vi "JSON text to Variant.vi"(6 "LVClass Serializer":refnum<class "JSONtext LVClass Serializer.lvclass">, 8 "error in (no error)":errorcluster, 9 "Data Type":variant, 10 "Offset":i32, 11 "JSON":string) -> (0 "error out":errorcluster, 1 "Variant out":variant)   [LabVIEW 2019, in "JSONtext.lvlib"]
doc: "Convert JSON to the Data Type entered, which may be a cluster or array."
uses:
  JSONtext.lvlib
  LVClass Serializer/JSONtext LVClass Serializer.lvclass
  <vilib>/Utility/Data Type/Type Definitions/Data Type.ctl
  Parsing/Advance past Line Ending.vi
  support/Get String.vi
  support/Get Timestamp.vi
  support/Get I32.vi
  support/Get I64.vi
  support/Get U32.vi
  support/Get U64.vi
  support/Get Boolean.vi
  support/Get DBL.vi
  support/Get SGL.vi
  support/Unescape JSON string.vi
  support/quote and escape json string 2.vi
  Parsing/Advance past whitespace and comma.vi
  Parsing/Advance past next JSON Value (inlined COPY).vi
  Parsing/Advance past Item Name.vi
  Base64/base64url Decode.vi
  Parsing/Advance past String.vi
  support/Get Number Text.vi
  Parsing/NaN or null to Integer ERROR.vi
  Parsing/Advance past Number.vi
  <vilib>/Utility/error.llb/Error Cluster From Error Code.vi
  <vilib>/Utility/Data Type/Get Refnum Information.vi
  support/Error Cluster From Code.vi
  JDP Science Common Utilities/Timestamp/Text to Timestamp.vi
  <vilib>/Utility/Data Type/Get Numeric Information.vi
  Parsing/Advance past Object.vi
  Parsing/Parsing Error.vi
  <vilib>/Utility/Data Type/NI_Data Type.lvlib
  JDP Science Common Utilities/JDP Utility.lvlib
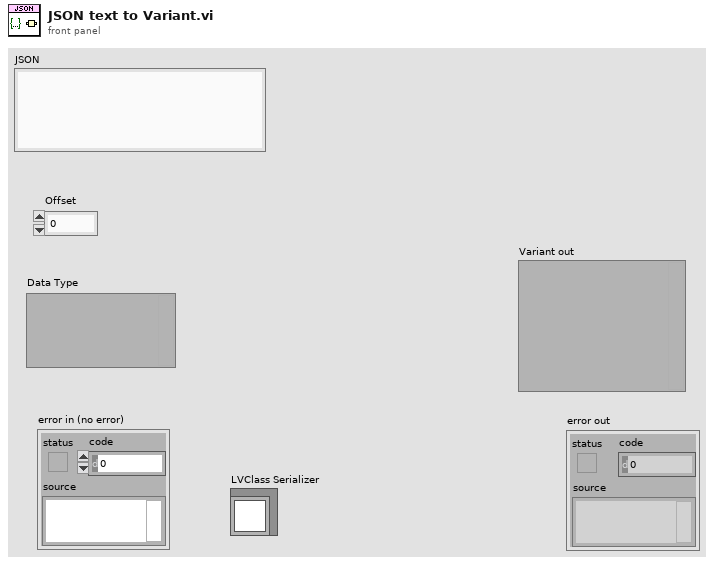
[diagram p1: front panel]
types:
  T1 = typedef "NI_Data Type.lvlib/Data Type.ctl" = enum8{"Invalid Type", "Void", "I8", "I16", "I32", "I64", "U8", "U16", "U32", "U64", "Single Float", "Double Float", "Extended Float", "Single Complex", "Double Complex", "Extended Complex", "Enum U8", "Enum U16", "Enum U32", "Enum U64", "Single Float With Unit", "Double Float With Unit", "Extended Float With Unit", "Single Complex with Unit", "Double Complex with Unit", "Extended Complex with Unit", "Boolean", "String", "Path", "Picture", "Tag", "Array", "Cluster", "Variant", "LV Variant", "Waveform", "Timestamp", "Digital Waveform", "Digital Data", "ExpressData", "Refnum", "External Data", "VI", "Poly VI", "LabVIEW Class Instance", "Fixed Point", "Set Collection", "Map Collection"}
  T2 = typedef "JSONtext.lvlib/Parsing State.ctl" = enum16{"Parser Error", "Object", "Array", "String", "Number/Other", "Leading Whitespace", "Object end", "Array end", "Value end"}
  T3 = typedef "JSONtext.lvlib/Tag Type.ctl" = enum16{"No Tag", "<JSON>", "<JOBJ>"}
  T4 = typedef "JSONtext.lvlib/JSON Value Type.ctl" = enum16{"Not a JSON Value", "JSON Object", "JSON Array", "String", "Number", "true", "false", "null"}
  T5 = typedef "JSONtext.lvlib/Found Items.ctl" = cluster{"Item offset":i32, "Offset past Item":i32, "Name offset":i32, "Offset past Name":i32, "Found":bool, "Item Type":T2, "Item Index":i32, "Start Offset":i32, "Comma Needed For Insert":bool}
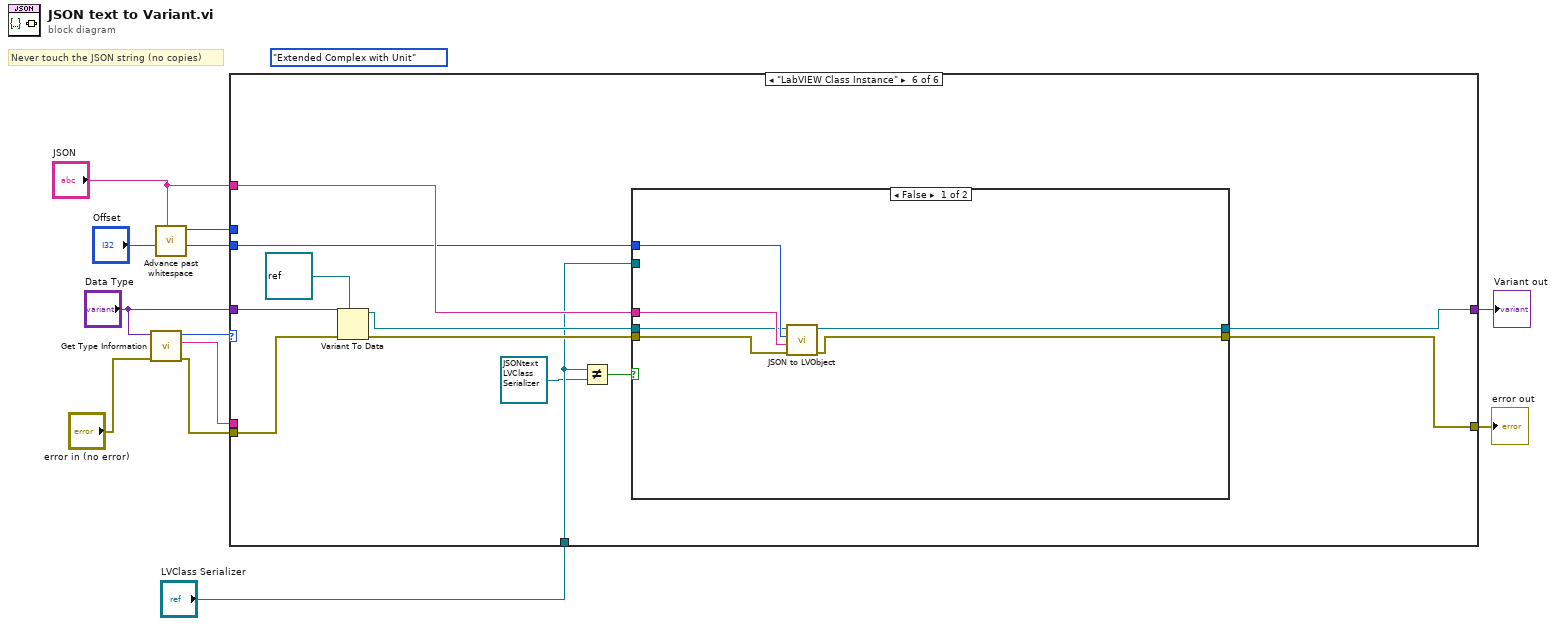
[diagram p0: block diagram]
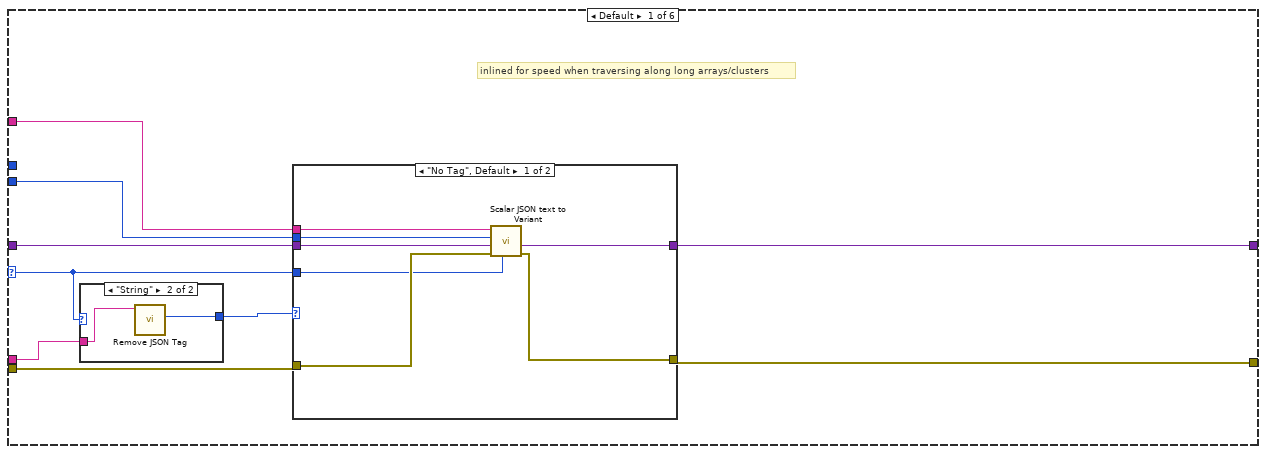
[diagram p2: hidden frame]
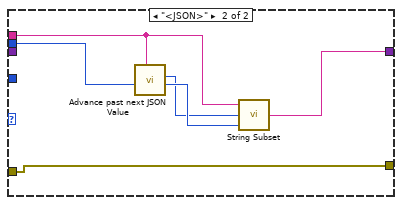
[diagram p3: hidden frame]
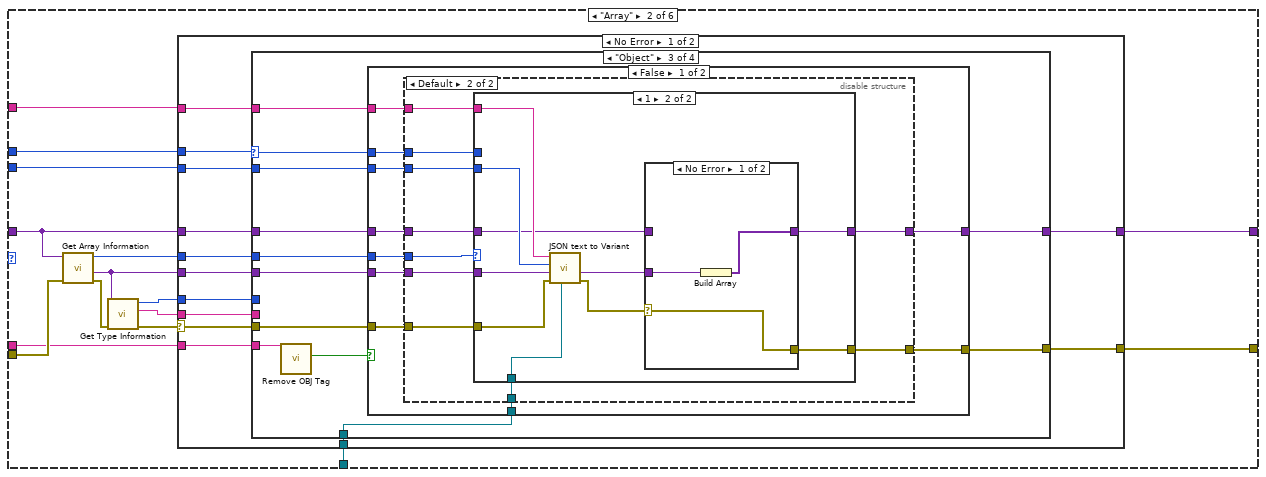
[diagram p5: hidden frame]
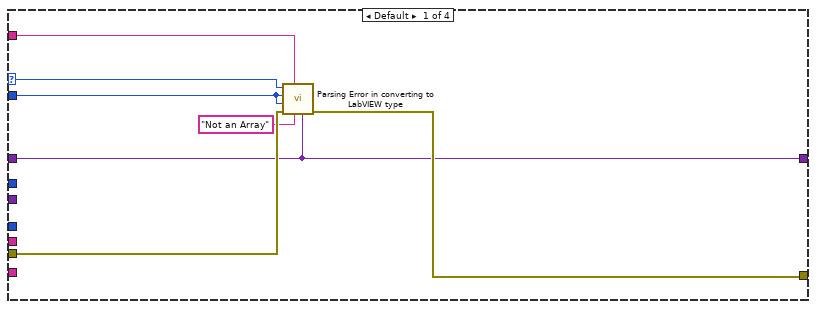
[diagram p6: hidden frame]
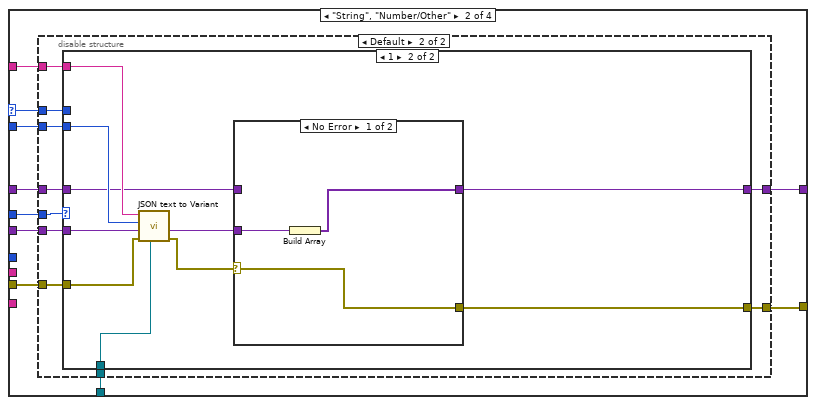
[diagram p7: hidden frame]
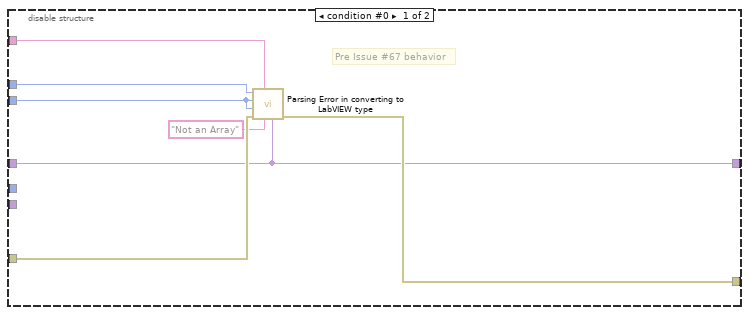
[diagram p8: hidden frame]
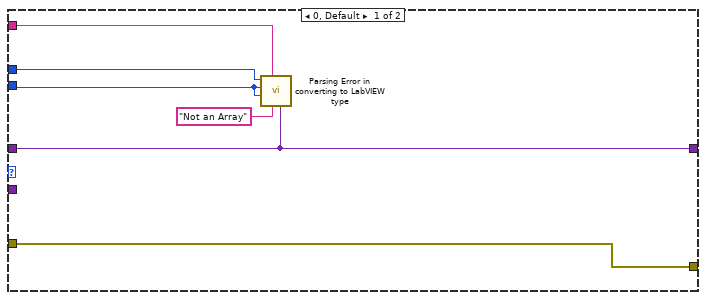
[diagram p9: hidden frame]
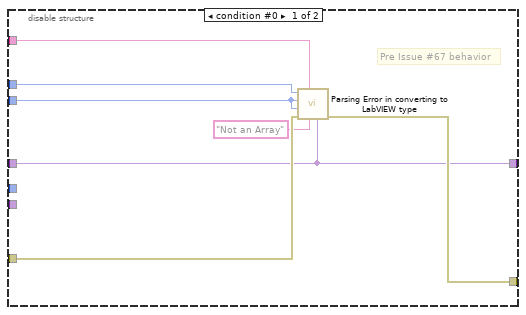
[diagram p11: hidden frame]
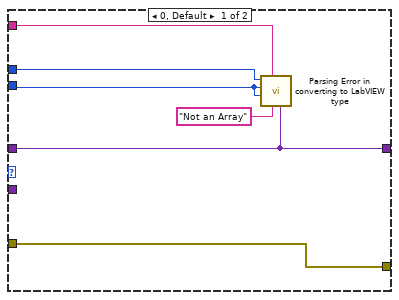
[diagram p12: hidden frame]
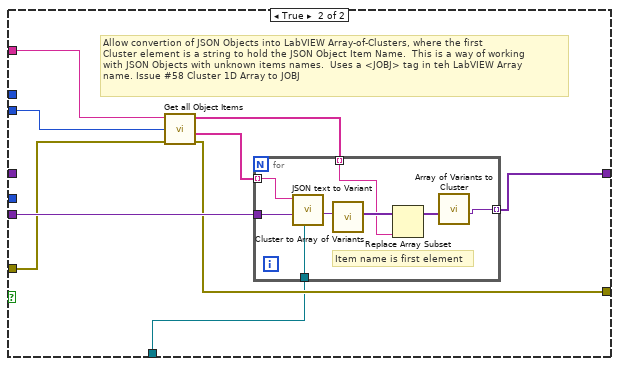
[diagram p14: hidden frame]
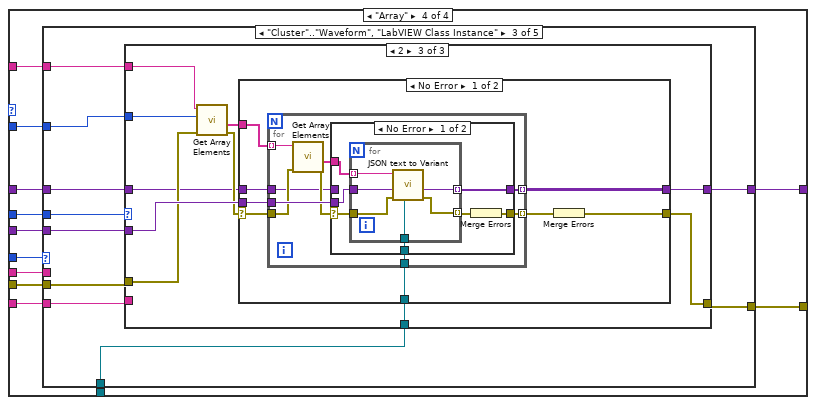
[diagram p15: hidden frame]
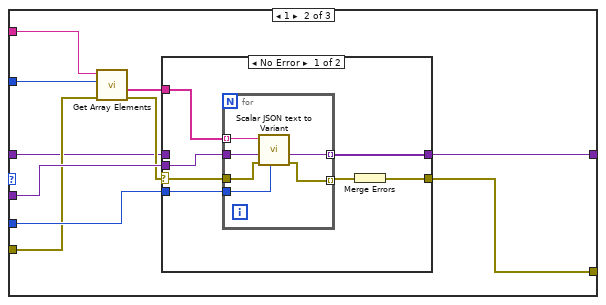
[diagram p18: hidden frame]
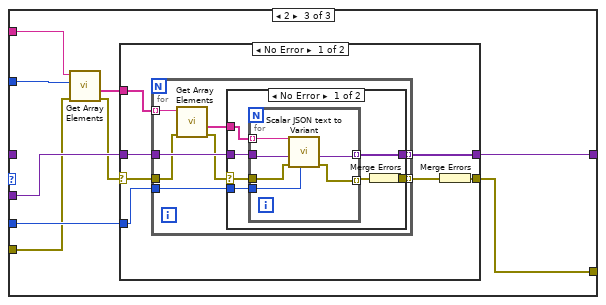
[diagram p20: hidden frame]
diagram:
  (unwired) Data_Type."Extended Complex with Unit" ("Type")
  # "Never touch the JSON string (no copies)"
  n1 = call <vilib>:"Get Type Information.vi"("error in (no error)"="error in (no error)", "variant"="Data Type") -> ("error out"=w8:errorcluster, "name"=w2:string, "type"=w12:T1)  [unwired: 5 in, 2 out]
  n2 = call "Advance past whitespace.vi"("JSON"="JSON", "Offset"="Offset") -> ("Offset of first non-whitespace"=w5:i32, "Parser State"=w3:T2)  [unwired: 7 in, 1 out]
  n3 = case shown="\"LabVIEW Class Instance\"" w12 {
    selector: w12 -> [w14 _ _ _ _ _]
    tunnel: "Data Type" -> [w21 w44 w586 w595 w795 w806]
    tunnel: "JSON" -> [w19 w42 w579 w591 w790 w807]
    tunnel: [w16 w48 w576 w593 w787 w800] -> w9
    tunnel: w8 -> [w17 w51 w585 w594 w794 w804]
    tunnel: w5 -> [w18 w40 w578 w592 w789 w799]
    tunnel: [w20 w47 w569 w588 w792 w801] -> w7
    tunnel: w3 -> [_ w38 _ _ _ _]
    tunnel: w2 -> [w15 w41 _ _ _ _]
    tunnel: "LVClass Serializer" -> [_ w37 w568 w587 w785 w798]
    frame Default {
      # "inlined for speed when traversing along long arrays/clusters"
      n4 = case shown="\"String\"" w14 {
        tunnel: w15 -> [_ w36]
        tunnel: [_ w35] -> w13
        frame "Invalid Type", Default {
        }
        frame "String" {
          n5 = call "Remove JSON Tag.vi"("Name"=w36) -> ("Tag"=w35:T3)  [unwired: 9 in, 1 out]
        }
      }
      n6 = case shown="\"No Tag\", Default" w13 {
        tunnel: w21 -> [w28 _]
        tunnel: [w27 w30] -> w20
        tunnel: w19 -> [w26 w31]
        tunnel: w18 -> [w25 w34]
        tunnel: w17 -> [w24 w29]
        tunnel: [w23 w29] -> w16
        tunnel: w14 -> [w22 _]
        frame "No Tag", Default {
          n7 = call "Scalar JSON text to Variant.vi"("Type"=w22, "error in (no error)"=w24, "Variant (Data Type)"=w28, "Offset"=w25, "JSON"=w26) -> ("error out"=w23:errorcluster, "Variant out"=w27:variant)  [unwired: 5 in]
        }
        frame "<JSON>" {
          n8 = call "Advance past next JSON Value.vi"("JSON"=w31, "Offset"=w34) -> ("Offset out"=w33:i32, "Value start"=w32:i32)  [unwired: 7 in, 1 out]
          n9 = call "String Subset.vi"("Offset past End"=w33, "Start offset"=w32, "JSON"=w31) -> ("substring"=w30:string)  [unwired: 2 in]
        }
      }
    }
    frame "Array" {
      n10 = call <vilib>:"Get Array Information.vi"("error in (no error)"=w51, "variant"=w44) -> ("error out"=w50:errorcluster, "array element data type"=w43:variant, "number of dimensions"=w45:i32)  [unwired: 6 in, 1 out]
      n11 = call <vilib>:"Get Type Information.vi"("error in (no error)"=w50, "variant"=w43) -> ("error out"=w49:errorcluster, "name"=w39:string, "type"=w46:T1)  [unwired: 5 in, 2 out]
      n12 = case shown="No Error" w49 {
        selector: w49 -> [w64 w567]
        tunnel: [w63 w567] -> w48
        tunnel: [w62 w566] -> w47
        tunnel: w46 -> [w61 _]
        tunnel: w45 -> [w60 _]
        tunnel: w44 -> [w59 w566]
        tunnel: w43 -> [w58 _]
        tunnel: w42 -> [w57 _]
        tunnel: w41 -> [w56 _]
        tunnel: w40 -> [w55 _]
        tunnel: w39 -> [w54 _]
        tunnel: w38 -> [w53 _]
        tunnel: w37 -> [w52 _]
        frame No Error {
          n13 = case shown="\"Object\"" w53 {
            selector: w53 -> [w69 w79 w129 _]
            tunnel: w64 -> [w68 w78 w128 w208]
            tunnel: [w67 w77 w127 w207] -> w63
            tunnel: [w66 w74 w124 w206] -> w62
            tunnel: w61 -> [_ _ _ w205]
            tunnel: w60 -> [_ w73 w123 w204]
            tunnel: w59 -> [w66 w76 w126 w203]
            tunnel: w58 -> [_ w75 w125 w202]
            tunnel: w57 -> [w71 w81 w131 w201]
            tunnel: w56 -> [_ _ w121 w200]
            tunnel: w55 -> [w70 w80 w130 w199]
            tunnel: w54 -> [_ _ _ w198]
            tunnel: w52 -> [_ w72 w122 w197]
            frame Default {
              n14 = call "Parsing Error in converting to LabVIEW type.vi"("LV Type"=w66, "initial string"="Not an Array", "JSON"=w71, "error in (no error)"=w68, "Offset past match"=w70, "Value start"=w70, "State"=w69) -> ("error out"=w67:errorcluster)  [unwired: 4 in]
            }
            frame "String", "Number/Other" {
              n15 = disable-structure shown="Default" {
                disable-tunnel: w81 -> [w88 w97]
                disable-tunnel: w80 -> [w87 w96]
                disable-tunnel: w79 -> [w86 w90]
                disable-tunnel: w78 -> [w85 w95]
                disable-tunnel: [w84 w92] -> w77
                disable-tunnel: w76 -> [w82 w93]
                disable-tunnel: w75 -> [_ w98]
                disable-tunnel: [w82 w94] -> w74
                disable-tunnel: w73 -> [_ w91]
                disable-tunnel: w72 -> [_ w89]
                frame condition #0 {
                  # "Pre Issue #67 behavior"
                  n16 = call "Parsing Error in converting to LabVIEW type.vi"("LV Type"=w82, "initial string"="Not an Array", "JSON"=w88, "error in (no error)"=w85, "Offset past match"=w87, "Value start"=w87, "State"=w86) -> ("error out"=w84:errorcluster)  [unwired: 4 in]
                }
                frame condition #1 (active) {
                  n17 = case shown="1" w91 {
                    tunnel: w98 -> [_ w114]
                    tunnel: w97 -> [w103 w113]
                    tunnel: w96 -> [w101 w112]
                    tunnel: w95 -> [w99 w110]
                    tunnel: [w100 w108] -> w94
                    tunnel: w93 -> [w100 w107]
                    tunnel: [w99 w106] -> w92
                    tunnel: w90 -> [w102 _]
                    tunnel: w89 -> [_ w105]
                    frame 0, Default {
                      n18 = call "Parsing Error in converting to LabVIEW type.vi"("LV Type"=w100, "initial string"="Not an Array", "JSON"=w103, "Offset past match"=w101, "Value start"=w101, "State"=w102) -> ()  [unwired: 5 in, 1 out]
                    }
                    frame 1 {
                      n19 = call "JSON text to Variant.vi"("LVClass Serializer"=w105, "error in (no error)"=w110, "Data Type"=w114, "Offset"=w112, "JSON"=w113) -> ("error out"=w109:errorcluster, "Variant out"=w111:variant)  [unwired: 5 in]
                      n20 = case shown="No Error" w109 {
                        selector: w109 -> [w115 w118]
                        tunnel: w111 -> [w117 _]
                        tunnel: [w116 w119] -> w108
                        tunnel: w107 -> [_ w119]
                        tunnel: [w115 w118] -> w106
                        frame No Error {
                          n21 = Build Array(w117) -> (w116:variant[])
                        }
                        frame Error {
                        }
                      }
                    }
                  }
                }
              }
            }
            frame "Object" {
              n22 = call "Remove OBJ Tag.vi"("Name"=w121) -> ("tagged as Item Name in JSON Objects"=w120:bool)  [unwired: 9 in, 1 out]
              n23 = case shown="False" w120 {
                tunnel: w131 -> [w141 w186]
                tunnel: w130 -> [w140 w180]
                tunnel: w129 -> [w139 _]
                tunnel: w128 -> [w138 w187]
                tunnel: [w137 w184] -> w127
                tunnel: w126 -> [w136 _]
                tunnel: w125 -> [w135 w188]
                tunnel: [w134 w185] -> w124
                tunnel: w123 -> [w133 _]
                tunnel: w122 -> [w132 w183]
                frame False {
                  n24 = disable-structure shown="Default" {
                    disable-tunnel: w141 -> [w148 w157]
                    disable-tunnel: w140 -> [w147 w156]
                    disable-tunnel: w139 -> [w146 w150]
                    disable-tunnel: w138 -> [w145 w155]
                    disable-tunnel: [w144 w152] -> w137
                    disable-tunnel: w136 -> [w142 w153]
                    disable-tunnel: w135 -> [_ w158]
                    disable-tunnel: [w142 w154] -> w134
                    disable-tunnel: w133 -> [_ w151]
                    disable-tunnel: w132 -> [_ w149]
                    frame condition #0 {
                      # "Pre Issue #67 behavior"
                      n25 = call "Parsing Error in converting to LabVIEW type.vi"("LV Type"=w142, "initial string"="Not an Array", "JSON"=w148, "error in (no error)"=w145, "Offset past match"=w147, "Value start"=w147, "State"=w146) -> ("error out"=w144:errorcluster)  [unwired: 4 in]
                    }
                    frame condition #1 (active) {
                      n26 = case shown="1" w151 {
                        tunnel: w158 -> [_ w174]
                        tunnel: w157 -> [w163 w173]
                        tunnel: w156 -> [w161 w172]
                        tunnel: w155 -> [w159 w170]
                        tunnel: [w160 w168] -> w154
                        tunnel: w153 -> [w160 w167]
                        tunnel: [w159 w166] -> w152
                        tunnel: w150 -> [w162 _]
                        tunnel: w149 -> [_ w165]
                        frame 0, Default {
                          n27 = call "Parsing Error in converting to LabVIEW type.vi"("LV Type"=w160, "initial string"="Not an Array", "JSON"=w163, "Offset past match"=w161, "Value start"=w161, "State"=w162) -> ()  [unwired: 5 in, 1 out]
                        }
                        frame 1 {
                          n28 = call "JSON text to Variant.vi"("LVClass Serializer"=w165, "error in (no error)"=w170, "Data Type"=w174, "Offset"=w172, "JSON"=w173) -> ("error out"=w169:errorcluster, "Variant out"=w171:variant)  [unwired: 5 in]
                          n29 = case shown="No Error" w169 {
                            selector: w169 -> [w175 w178]
                            tunnel: w171 -> [w177 _]
                            tunnel: [w176 w179] -> w168
                            tunnel: w167 -> [_ w179]
                            tunnel: [w175 w178] -> w166
                            frame No Error {
                              n30 = Build Array(w177) -> (w176:variant[])
                            }
                            frame Error {
                            }
                          }
                        }
                      }
                    }
                  }
                }
                frame True {
                  # "Allow convertion of JSON Objects into LabVIEW Array-of-Clusters, where the first\nCluster element is a string to hold the JSON Object Item Name.  This is a way of working\nwith JSON Objects with unknown items names.  Uses a <JOBJ> tag in teh LabVIEW Array\nname. Issue #58 Cluster 1D Array to JOBJ"
                  n31 = call "Get all Object Items.vi"("error in (no error)"=w187, "Offset"=w180, "JSON"=w186) -> ("error out"=w184:errorcluster, "<JSON>"=w182:string[], "Item Names"=w181:string[])  [unwired: 5 in, 1 out]
                  n32 = for {
                    tunnel: w182 -> [w196] mode=indexing
                    tunnel: w188 -> [w195]
                    tunnel: w181 -> [w191] mode=indexing
                    tunnel: [w190] -> w185 mode=indexing
                    tunnel: w183 -> [w189]
                    # "Item name is first element"
                    n33 = call "JSON text to Variant.vi"("LVClass Serializer"=w189, "Data Type"=w195, "JSON"=w196) -> ("Variant out"=w193:variant)  [unwired: 7 in, 1 out]
                    n34 = call "Cluster to Array of Variants.vi"("Cluster"=w193) -> ("Array of Cluster Elements"=w192:variant[])  [unwired: 10 in]
                    n35 = Replace Array Subset(array=w192, new element=w191) -> (w194:variant[])  [unwired: 1 in]
                    n36 = call "Array of Variants to Cluster.vi"("Array of Variants"=w194) -> ("Cluster of Variants"=w190:variant)  [unwired: 10 in]
                  }
                }
              }
            }
            frame "Array" {
              n37 = case shown="\"Cluster\"..\"Waveform\", \"LabVIEW Class Instance\"" w205 {
                selector: w205 -> [_ w211 _ w375 _]
                tunnel: w201 -> [_ w215 w293 w373 w503]
                tunnel: w208 -> [w209 w218 w296 w380 w502]
                tunnel: [w209 w219 w297 w379 w501] -> w207
                tunnel: [w210 w216 w294 w378 w500] -> w206
                tunnel: w204 -> [_ w214 w292 w377 w499]
                tunnel: w203 -> [w210 w213 w291 w376 w498]
                tunnel: w202 -> [_ w217 w295 _ _]
                tunnel: w199 -> [_ w212 w290 w372 w496]
                tunnel: w200 -> [_ _ w289 _ w497]
                tunnel: w198 -> [_ _ _ _ w495]
                tunnel: w197 -> [_ _ w288 _ _]
                frame "Invalid Type" {
                }
                frame Default {
                  # "Scaler type (so we are using the inlined function"
                  n38 = case shown="0, Default" w214 {
                    tunnel: [w220 w231 w250] -> w219
                    tunnel: w218 -> [w220 w224 w248]
                    tunnel: w217 -> [_ w230 w255]
                    tunnel: [w221 w228 w253] -> w216
                    tunnel: w212 -> [_ w227 w252]
                    tunnel: w215 -> [_ w226 w251]
                    tunnel: w213 -> [w221 w222 _]
                    tunnel: w211 -> [_ w225 w249]
                    frame 0, Default {
                    }
                    frame 1 {
                      n39 = call "Get Array Elements.vi"("error in (no error)"=w224, "Offset"=w227, "JSON"=w226) -> ("error out"=w223:errorcluster, "<JSON>"=w229:string[])  [unwired: 6 in, 1 out]
                      n40 = case shown="No Error" w223 {
                        selector: w223 -> [w232 w245]
                        tunnel: [w237 w245] -> w231
                        tunnel: w230 -> [w236 _]
                        tunnel: w229 -> [w235 _]
                        tunnel: [w234 w246] -> w228
                        tunnel: w225 -> [w233 _]
                        tunnel: w222 -> [_ w246]
                        frame No Error {
                          n41 = for {
                            tunnel: w236 -> [w243]
                            tunnel: w232 -> [w241]
                            tunnel: [w240] -> w238 mode=indexing
                            tunnel: [w242] -> w234 mode=indexing
                            tunnel: w235 -> [w244] mode=indexing
                            tunnel: w233 -> [w239]
                            n42 = call "Scalar JSON text to Variant.vi"("Type"=w239, "error in (no error)"=w241, "Variant (Data Type)"=w243, "JSON"=w244) -> ("error out"=w240:errorcluster, "Variant out"=w242:variant)  [unwired: 6 in]
                          }
                          n43 = Merge Errors(w238) -> (w237:errorcluster)
                        }
                        frame Error {
                        }
                      }
                    }
                    frame 2 {
                      n44 = call "Get Array Elements.vi"("error in (no error)"=w248, "Offset"=w252, "JSON"=w251) -> ("error out"=w247:errorcluster, "<JSON>"=w254:string[])  [unwired: 6 in, 1 out]
                      n45 = case shown="No Error" w247 {
                        selector: w247 -> [w256 w287]
                        tunnel: w255 -> [w261 w286]
                        tunnel: w254 -> [w260 _]
                        tunnel: [w259 w286] -> w253
                        tunnel: [w258 w287] -> w250
                        tunnel: w249 -> [w257 _]
                        frame No Error {
                          n46 = for {
                            tunnel: [w270] -> w262 mode=indexing
                            tunnel: w256 -> [w264]
                            tunnel: w261 -> [w269]
                            tunnel: w260 -> [w267] mode=indexing
                            tunnel: [w268] -> w259 mode=indexing
                            tunnel: w257 -> [w265]
                            n47 = call "Get Array Elements.vi"("error in (no error)"=w264, "JSON"=w267) -> ("error out"=w263:errorcluster, "<JSON>"=w266:string[])  [unwired: 7 in, 1 out]
                            n48 = case shown="No Error" w263 {
                              selector: w263 -> [w271 w284]
                              tunnel: [w276 w284] -> w270
                              tunnel: w269 -> [w275 w285]
                              tunnel: [w274 w285] -> w268
                              tunnel: w266 -> [w273 _]
                              tunnel: w265 -> [w272 _]
                              frame No Error {
                                n49 = for {
                                tunnel: w275 -> [w279]
                                tunnel: w271 -> [w280]
                                tunnel: [w281] -> w277 mode=indexing
                                tunnel: [w282] -> w274 mode=indexing
                                tunnel: w273 -> [w283] mode=indexing
                                tunnel: w272 -> [w278]
                                n50 = call "Scalar JSON text to Variant.vi"("Type"=w278, "error in (no error)"=w280, "Variant (Data Type)"=w279, "JSON"=w283) -> ("error out"=w281:errorcluster, "Variant out"=w282:variant)  [unwired: 6 in]
                                }
                                n51 = Merge Errors(w277) -> (w276:errorcluster)
                              }
                              frame Error {
                              }
                            }
                          }
                          n52 = Merge Errors(w262) -> (w258:errorcluster)
                        }
                        frame Error {
                        }
                      }
                    }
                  }
                }
                frame "Cluster".."Waveform", "LabVIEW Class Instance" {
                  n53 = case shown="2" w292 {
                    tunnel: [w298 w309 w329] -> w297
                    tunnel: w296 -> [w298 w308 w328]
                    tunnel: w295 -> [_ w307 w334]
                    tunnel: [w299 w306 w332] -> w294
                    tunnel: w290 -> [_ w304 w331]
                    tunnel: w293 -> [_ w305 w330]
                    tunnel: w291 -> [w299 w303 w326]
                    tunnel: w289 -> [_ _ _]
                    tunnel: w288 -> [_ w302 w325]
                    frame 0, Default {
                    }
                    frame 1 {
                      n54 = call "Get Array Elements.vi"("error in (no error)"=w308, "Offset"=w304, "JSON"=w305) -> ("error out"=w300:errorcluster, "<JSON>"=w301:string[])  [unwired: 6 in, 1 out]
                      n55 = case shown="No Error" w300 {
                        selector: w300 -> [w311 w324]
                        tunnel: [w315 w324] -> w309
                        tunnel: w307 -> [w314 _]
                        tunnel: [w313 w323] -> w306
                        tunnel: w301 -> [w312 _]
                        tunnel: w303 -> [_ w323]
                        tunnel: w302 -> [w310 _]
                        frame No Error {
                          n56 = for {
                            tunnel: w314 -> [w322]
                            tunnel: w311 -> [w321]
                            tunnel: [w320] -> w316 mode=indexing
                            tunnel: [w319] -> w313 mode=indexing
                            tunnel: w312 -> [w318] mode=indexing
                            tunnel: w310 -> [w317]
                            n57 = call "JSON text to Variant.vi"("LVClass Serializer"=w317, "error in (no error)"=w321, "Data Type"=w322, "JSON"=w318) -> ("error out"=w320:errorcluster, "Variant out"=w319:variant)  [unwired: 6 in]
                          }
                          n58 = Merge Errors(w316) -> (w315:errorcluster)
                        }
                        frame Error {
                        }
                      }
                    }
                    frame 2 {
                      n59 = call "Get Array Elements.vi"("error in (no error)"=w328, "Offset"=w331, "JSON"=w330) -> ("error out"=w327:errorcluster, "<JSON>"=w333:string[])  [unwired: 6 in, 1 out]
                      n60 = case shown="No Error" w327 {
                        selector: w327 -> [w337 w369]
                        tunnel: w334 -> [w341 _]
                        tunnel: w333 -> [w340 _]
                        tunnel: [w339 w368] -> w332
                        tunnel: [w338 w369] -> w329
                        tunnel: w326 -> [w336 w368]
                        tunnel: w325 -> [w335 _]
                        frame No Error {
                          n61 = for {
                            tunnel: [w351] -> w342 mode=indexing
                            tunnel: w337 -> [w346]
                            tunnel: w341 -> [w350]
                            tunnel: w340 -> [w348] mode=indexing
                            tunnel: [w349] -> w339 mode=indexing
                            tunnel: w336 -> [w344]
                            tunnel: w335 -> [w343]
                            n62 = call "Get Array Elements.vi"("error in (no error)"=w346, "JSON"=w348) -> ("error out"=w345:errorcluster, "<JSON>"=w347:string[])  [unwired: 7 in, 1 out]
                            n63 = case shown="No Error" w345 {
                              selector: w345 -> [w353 w367]
                              tunnel: [w357 w367] -> w351
                              tunnel: w350 -> [w356 w365]
                              tunnel: [w355 w366] -> w349
                              tunnel: w347 -> [w354 _]
                              tunnel: w344 -> [_ _]
                              tunnel: w343 -> [w352 _]
                              frame No Error {
                                n64 = for {
                                tunnel: w356 -> [w364]
                                tunnel: w353 -> [w363]
                                tunnel: [w362] -> w358 mode=indexing
                                tunnel: [w361] -> w355 mode=indexing
                                tunnel: w354 -> [w360] mode=indexing
                                tunnel: w352 -> [w359]
                                n65 = call "JSON text to Variant.vi"("LVClass Serializer"=w359, "error in (no error)"=w363, "Data Type"=w364, "JSON"=w360) -> ("error out"=w362:errorcluster, "Variant out"=w361:variant)  [unwired: 6 in]
                                }
                                n66 = Merge Errors(w358) -> (w357:errorcluster)
                              }
                              frame Error {
                                n67 = Build Array(w365) -> (w366:variant[])
                              }
                            }
                          }
                          n68 = Merge Errors(w342) -> (w338:errorcluster)
                        }
                        frame Error {
                        }
                      }
                    }
                  }
                }
                frame "I8".."Extended Complex", "Single Float With Unit".."Extended Float With Unit" {
                  # "Use LV JSON primative for speed"
                  n69 = call "Advance past Array.vi"("JSON"=w373, "Offset"=w372) -> ("Offset past Array"=w374:i32, "Empty Array"=w370:bool, "Array Start"=w371:i32)  [unwired: 6 in, 1 out]
                  n70 = case shown="False" w370 {
                    tunnel: w380 -> [w390 w493]
                    tunnel: [w389 w493] -> w379
                    tunnel: [w388 w492] -> w378
                    tunnel: w377 -> [w387 _]
                    tunnel: w376 -> [w386 w492]
                    tunnel: w375 -> [w384 _]
                    tunnel: w374 -> [w383 _]
                    tunnel: w373 -> [w382 _]
                    tunnel: w371 -> [w381 _]
                    frame False {
                      n71 = call "String Subset.vi"("Offset past End"=w383, "Start offset"=w381, "JSON"=w382) -> ("substring"=w385:string)  [unwired: 2 in]
                      n72 = case shown="0, Default" w387 {
                        tunnel: w385 -> [_ w398 w431 w464]
                        tunnel: w390 -> [w391 w397 w430 w463]
                        tunnel: [w391 w396 w429 w462] -> w389
                        tunnel: [w392 w394 w427 w460] -> w388
                        tunnel: w386 -> [w392 w393 w426 w459]
                        tunnel: w384 -> [_ w395 w428 w461]
                        frame 0, Default {
                        }
                        frame 1 {
                          n73 = case shown="\"I8\"..\"I32\"" w395 {
                            tunnel: w398 -> [_ w405 w410 w415 w420 w425]
                            tunnel: w397 -> [w399 w403 w408 w413 w418 w423]
                            tunnel: [w399 w402 w407 w412 w417 w422] -> w396
                            tunnel: [w400 w401 w406 w411 w416 w421] -> w394
                            tunnel: w393 -> [w400 _ _ _ _ _]
                            frame "Invalid Type", Default {
                            }
                            frame "Single Float".."Extended Float", "Single Float With Unit".."Extended Float With Unit" {
                              n74 = Unflatten From JSON(JSON string=w405, type and defaults=dbl[] [], error in (no error)=w403) -> (value=w401:dbl[], error out=w402:errorcluster)  [unwired: 4 in]
                            }
                            frame "U8".."U32" {
                              n75 = Unflatten From JSON(JSON string=w410, type and defaults=u32[] [], error in (no error)=w408) -> (value=w406:u32[], error out=w407:errorcluster)  [unwired: 4 in]
                            }
                            frame "U64" {
                              n76 = Unflatten From JSON(JSON string=w415, type and defaults=u64[] [], error in (no error)=w413) -> (value=w411:u64[], error out=w412:errorcluster)  [unwired: 4 in]
                            }
                            frame "I8".."I32" {
                              n77 = Unflatten From JSON(JSON string=w420, type and defaults=i32[] [], error in (no error)=w418) -> (value=w416:i32[], error out=w417:errorcluster)  [unwired: 4 in]
                            }
                            frame "I64" {
                              n78 = Unflatten From JSON(JSON string=w425, type and defaults=i64[] [], error in (no error)=w423) -> (value=w421:i64[], error out=w422:errorcluster)  [unwired: 4 in]
                            }
                          }
                        }
                        frame 2 {
                          n79 = case shown="\"Single Float\"..\"Extended Float\", \"Single Float With Unit\"..\"Extended Float With Unit\"" w428 {
                            tunnel: w431 -> [_ w438 w443 w448 w453 w458]
                            tunnel: w430 -> [w432 w436 w441 w446 w451 w456]
                            tunnel: [w432 w435 w440 w445 w450 w455] -> w429
                            tunnel: [w433 w434 w439 w444 w449 w454] -> w427
                            tunnel: w426 -> [w433 _ _ _ _ _]
                            frame "Invalid Type", Default {
                            }
                            frame "Single Float".."Extended Float", "Single Float With Unit".."Extended Float With Unit" {
                              n80 = Unflatten From JSON(JSON string=w438, type and defaults=dbl[][] [], error in (no error)=w436) -> (value=w434:dbl[][], error out=w435:errorcluster)  [unwired: 4 in]
                            }
                            frame "U8".."U32" {
                              n81 = Unflatten From JSON(JSON string=w443, type and defaults=u32[][] [], error in (no error)=w441) -> (value=w439:u32[][], error out=w440:errorcluster)  [unwired: 4 in]
                            }
                            frame "U64" {
                              n82 = Unflatten From JSON(JSON string=w448, type and defaults=u64[][] [], error in (no error)=w446) -> (value=w444:u64[][], error out=w445:errorcluster)  [unwired: 4 in]
                            }
                            frame "I8".."I32" {
                              n83 = Unflatten From JSON(JSON string=w453, type and defaults=i32[][] [], error in (no error)=w451) -> (value=w449:i32[][], error out=w450:errorcluster)  [unwired: 4 in]
                            }
                            frame "I64" {
                              n84 = Unflatten From JSON(JSON string=w458, type and defaults=i64[][] [], error in (no error)=w456) -> (value=w454:i64[][], error out=w455:errorcluster)  [unwired: 4 in]
                            }
                          }
                        }
                        frame 3 {
                          n85 = case shown="\"I8\"..\"I32\"" w461 {
                            tunnel: w464 -> [_ w471 w476 w481 w486 w491]
                            tunnel: w463 -> [w465 w469 w474 w479 w484 w489]
                            tunnel: [w465 w468 w473 w478 w483 w488] -> w462
                            tunnel: [w466 w467 w472 w477 w482 w487] -> w460
                            tunnel: w459 -> [w466 _ _ _ _ _]
                            frame "Invalid Type", Default {
                            }
                            frame "Single Float".."Extended Float", "Single Float With Unit".."Extended Float With Unit" {
                              n86 = Unflatten From JSON(JSON string=w471, type and defaults=dbl[][][] [], error in (no error)=w469) -> (value=w467:dbl[][][], error out=w468:errorcluster)  [unwired: 4 in]
                            }
                            frame "U8".."U32" {
                              n87 = Unflatten From JSON(JSON string=w476, type and defaults=u32[][][] [], error in (no error)=w474) -> (value=w472:u32[][][], error out=w473:errorcluster)  [unwired: 4 in]
                            }
                            frame "U64" {
                              n88 = Unflatten From JSON(JSON string=w481, type and defaults=u64[][][] [], error in (no error)=w479) -> (value=w477:u64[][][], error out=w478:errorcluster)  [unwired: 4 in]
                            }
                            frame "I8".."I32" {
                              n89 = Unflatten From JSON(JSON string=w486, type and defaults=i32[][][] [], error in (no error)=w484) -> (value=w482:i32[][][], error out=w483:errorcluster)  [unwired: 4 in]
                            }
                            frame "I64" {
                              n90 = Unflatten From JSON(JSON string=w491, type and defaults=i64[][][] [], error in (no error)=w489) -> (value=w487:i64[][][], error out=w488:errorcluster)  [unwired: 4 in]
                            }
                          }
                        }
                      }
                    }
                    frame True {
                    }
                  }
                }
                frame "String" {
                  n91 = call "JSON Tags on Array.vi"("Array Name"=w497, "Element Name"=w495) -> ("Tag"=w494:T3)  [unwired: 9 in]
                  n92 = case shown="\"No Tag\", Default" w494 {
                    tunnel: w503 -> [w510 w547]
                    tunnel: w502 -> [w509 w546]
                    tunnel: [w508 w545] -> w501
                    tunnel: [w507 w544] -> w500
                    tunnel: w499 -> [w506 w543]
                    tunnel: w498 -> [w505 w542]
                    tunnel: w496 -> [w504 w541]
                    frame "No Tag", Default {
                      # "#ds issue #2 Can't use LV primative\nbecause it mishandles zero bytes."
                      n93 = case shown="1" w506 {
                        tunnel: w510 -> [_ w517 w525]
                        tunnel: w509 -> [w511 w514 w526]
                        tunnel: [w511 w515 w527] -> w508
                        tunnel: [w512 w516 w528] -> w507
                        tunnel: w505 -> [w512 _ _]
                        tunnel: w504 -> [_ w513 w524]
                        frame 0, Default {
                        }
                        frame 1 {
                          n94 = call "Get Array Elements.vi"("error in (no error)"=w514, "Offset"=w513, "JSON"=w517) -> ("error out"=w519:errorcluster, "<JSON>"=w518:string[])  [unwired: 6 in, 1 out]
                          n95 = for {
                            tunnel: w518 -> [w523] mode=indexing
                            tunnel: [w522] -> w516 mode=indexing
                            shift-right: [w521] -> w515
                            shift-left: w519 -> [w520]
                            n96 = call "Strip Quotes and Unescape.vi"("error in (no error)"=w520, "String"=w523) -> ("error out"=w521:errorcluster, "result string"=w522:string)  [unwired: 8 in]
                          }
                        }
                        frame 2 {
                          n97 = call "Get Array Elements.vi"("error in (no error)"=w526, "Offset"=w524, "JSON"=w525) -> ("error out"=w530:errorcluster, "<JSON>"=w529:string[])  [unwired: 6 in, 1 out]
                          n98 = for {
                            tunnel: w529 -> [w536] mode=indexing
                            tunnel: [w533] -> w528 mode=indexing
                            shift-right: [w532] -> w527
                            shift-left: w530 -> [w535]
                            n99 = call "Get Array Elements.vi"("error in (no error)"=w535, "JSON"=w536) -> ("error out"=w531:errorcluster, "<JSON>"=w534:string[])  [unwired: 7 in, 1 out]
                            n100 = for {
                              tunnel: w534 -> [w540] mode=indexing
                              tunnel: [w539] -> w533 mode=indexing
                              shift-right: [w538] -> w532
                              shift-left: w531 -> [w537]
                              n101 = call "Strip Quotes and Unescape.vi"("error in (no error)"=w537, "String"=w540) -> ("error out"=w538:errorcluster, "result string"=w539:string)  [unwired: 8 in]
                            }
                          }
                        }
                      }
                    }
                    frame "<JSON>" {
                      # "JSON text"
                      n102 = case shown="2" w543 {
                        tunnel: w547 -> [_ w554 w556]
                        tunnel: w546 -> [w548 w553 w557]
                        tunnel: [w548 w552 w558] -> w545
                        tunnel: [w549 w551 w559] -> w544
                        tunnel: w542 -> [w549 _ _]
                        tunnel: w541 -> [_ w550 w555]
                        frame 0, Default {
                        }
                        frame 1 {
                          n103 = call "Get Array Elements.vi"("error in (no error)"=w553, "Offset"=w550, "JSON"=w554) -> ("error out"=w552:errorcluster, "<JSON>"=w551:string[])  [unwired: 6 in, 1 out]
                        }
                        frame 2 {
                          n104 = call "Get Array Elements.vi"("error in (no error)"=w557, "Offset"=w555, "JSON"=w556) -> ("error out"=w561:errorcluster, "<JSON>"=w560:string[])  [unwired: 6 in, 1 out]
                          n105 = for {
                            tunnel: w560 -> [w565] mode=indexing
                            tunnel: [w562] -> w559 mode=indexing
                            shift-right: [w563] -> w558
                            shift-left: w561 -> [w564]
                            n106 = call "Get Array Elements.vi"("error in (no error)"=w564, "JSON"=w565) -> ("error out"=w563:errorcluster, "<JSON>"=w562:string[])  [unwired: 7 in, 1 out]
                          }
                        }
                      }
                    }
                  }
                }
              }
            }
          }
        }
        frame Error {
        }
      }
    }
    frame "Waveform" {
      # "Attributes not supported"
      n107 = Variant To Data(error in=w585, type=waveform(dbl) {"t0"=timestamp(0 s since 1904-01-01), "dt"=1.0, "Y"=[]} ("waveform"), Variant=w586) -> (data=w583:waveform(dbl), error out=w577:errorcluster)
      n108 = Unbundle By Name(w583) -> ("t0"=w582:timestamp, "dt"=w581:dbl, "Y"=w580:dbl[])  [unwired: 1 out]
      n109 = Bundle("t0"=w582, "dt"=w581, "Y"=w580) -> (w574:cluster{"t0":timestamp, "dt":dbl, "Y":dbl[]})  [unwired: 1 in]
      n110 = call "JSON text to Variant.vi"("LVClass Serializer"=w568, "error in (no error)"=w577, "Data Type"=w574, "Offset"=w578, "JSON"=w579) -> ("error out"=w576:errorcluster, "Variant out"=w575:variant)  [unwired: 5 in]
      n111 = Variant To Data(type=w574, Variant=w575) -> (data=w573:cluster{"t0":timestamp, "dt":dbl, "Y":dbl[]})  [unwired: 1 in, 1 out]
      n112 = Unbundle By Name(w573) -> ("t0"=w572:timestamp, "dt"=w571:dbl, "Y"=w570:dbl[])
      n113 = Bundle By Name("t0"=w572, "dt"=w571, "Y"=w570) -> (w569:waveform(dbl))  [unwired: 1 in]
    }
    frame "Cluster" {
      n114 = call "JSON type.vi"("Offset"=w592, "JSON"=w591) -> ("Item Offset"=w590:i32, "JSON Value Type"=w589:T4)  [unwired: 8 in]
      n115 = case shown="\"JSON Array\"" w589 {
        selector: w589 -> [w600 _ w714]
        tunnel: w595 -> [w597 w621 w724]
        tunnel: w594 -> [w596 w619 w722]
        tunnel: [w597 w608 w715] -> w588
        tunnel: [w598 w617 w721] -> w593
        tunnel: w591 -> [_ w614 w718]
        tunnel: w590 -> [_ w613 w717]
        tunnel: w587 -> [_ w603 w713]
        frame Default {
          # "Issue #65"
          n116 = Format Into String(w600) -> (resulting string=w599:string)  [unwired: 3 in, 1 out]
          n117 = call "Format Error.vi"("error code (402842)"=402844, "error in (no error)"=w596, "message part 2"=w599, "error message"="Cannot Get as a Cluster: " ("format string")) -> ("error out"=w598:errorcluster)  [unwired: 7 in]
        }
        frame "JSON Object" {
          n118 = Variant To Data(error in=w619, type=variant[] [], Variant=w621) -> (data=w615:variant[], error out=w616:errorcluster)
          n119 = for {
            tunnel: w615 -> [w708] mode=indexing
            tunnel: w616 -> [w707]
            tunnel: [w706] -> w612 mode=indexing
            tunnel: [w704] -> w609 mode=indexing
            tunnel: [w705] -> w611 mode=indexing
            tunnel: [w702] -> w610 mode=indexing
            n120 = call <vilib>:"Get Type Information.vi"("error in (no error)"=w707, "variant"=w708) -> ("error out"=w706:errorcluster, "name"=w703:string, "type"=w704:T1)  [unwired: 5 in, 2 out]
            n121 = case shown="\"String\", \"Array\"" w704 {
              tunnel: w703 -> [w709 w712]
              tunnel: [_ w711] -> w705
              tunnel: [w709 w710] -> w701
              frame Default {
              }
              frame "String", "Array" {
                n122 = call "Remove JSON Tag.vi"("Name"=w712) -> ("Tag"=w711:T3, "Name (tag stripped)"=w710:string)  [unwired: 9 in]
              }
            }
            n123 = call "Quote and Escape JSON string.vi"("Plain Text"=w701) -> ("<JSON>"=w702:string)  [unwired: 10 in]
          }
          n124 = call "Find Object Item Locations by Names.vi"("Insertion point if not found"=TRUE, "Item Names <JSON>"=w610, "error in (no error)"=w616, "Object Offset"=w613, "JSON"=w614) -> ("error out"=w604:errorcluster, "Items"=w606:T5[])  [unwired: 5 in]
          n125 = case shown="No Error" w604 {
            tunnel: [w630 w699] -> w607
            tunnel: [w629 w700] -> w618
            tunnel: w612 -> [w628 w699]
            tunnel: w606 -> [w627 _]
            tunnel: w611 -> [w626 _]
            tunnel: w609 -> [w625 _]
            tunnel: w615 -> [w624 w700]
            tunnel: w614 -> [w623 _]
            tunnel: w603 -> [w622 _]
            frame No Error {
              n126 = for {
                tunnel: w624 -> [w642] mode=indexing
                tunnel: w623 -> [w641]
                tunnel: [w640] -> w630 mode=indexing
                tunnel: [w639] -> w629 mode=indexing
                tunnel: w628 -> [w638] mode=indexing
                tunnel: w625 -> [w637] mode=indexing
                tunnel: w627 -> [w636] mode=indexing
                tunnel: w626 -> [w632] mode=indexing
                tunnel: w622 -> [w631]
                n127 = Unbundle By Name(w636) -> ("Found"=w635:bool, "Item offset"=w634:i32, "Offset past Item"=w633:i32)
                n128 = case shown="True" w635 {
                  tunnel: w641 -> [_ w654]
                  tunnel: w634 -> [_ w653]
                  tunnel: w642 -> [w644 w652]
                  tunnel: [w644 w648] -> w639
                  tunnel: w638 -> [w643 w651]
                  tunnel: [w643 w650] -> w640
                  tunnel: w637 -> [_ w649]
                  tunnel: w633 -> [_ w646]
                  tunnel: w632 -> [_ w647]
                  tunnel: w631 -> [_ w645]
                  frame False {
                  }
                  frame True {
                    n129 = case shown="\"<JSON>\"" w647 {
                      tunnel: w654 -> [w663 w686]
                      tunnel: w653 -> [w662 w685]
                      tunnel: w652 -> [w661 w679]
                      tunnel: w651 -> [w660 w681]
                      tunnel: [w659 w680] -> w650
                      tunnel: w649 -> [w656 w682]
                      tunnel: [w658 w683] -> w648
                      tunnel: w646 -> [_ w684]
                      tunnel: w645 -> [w655 w678]
                      frame "No Tag", Default {
                        n130 = call "Is Scaler Type.vi"("Type"=w656) -> ("Scaler Type"=w657:bool)  [unwired: 2 in]
                        n131 = case shown="False" w657 {
                          tunnel: w663 -> [w670 w677]
                          tunnel: w662 -> [w669 w676]
                          tunnel: [w668 w675] -> w658
                          tunnel: w661 -> [w666 w674]
                          tunnel: w660 -> [w665 w673]
                          tunnel: [w667 w672] -> w659
                          tunnel: w656 -> [w664 _]
                          tunnel: w655 -> [_ w671]
                          frame True {
                            n132 = call "Scalar JSON text to Variant.vi"("Type"=w664, "error in (no error)"=w665, "Variant (Data Type)"=w666, "Offset"=w669, "JSON"=w670) -> ("error out"=w667:errorcluster, "Variant out"=w668:variant)  [unwired: 5 in]
                          }
                          frame False {
                            n133 = call "JSON text to Variant.vi"("LVClass Serializer"=w671, "error in (no error)"=w673, "Data Type"=w674, "Offset"=w676, "JSON"=w677) -> ("error out"=w672:errorcluster, "Variant out"=w675:variant)  [unwired: 5 in]
                          }
                        }
                      }
                      frame "<JSON>" {
                        # "<JSON>"
                        n134 = case shown="\"Array\"" w682 {
                          tunnel: w686 -> [w693 w698]
                          tunnel: w685 -> [w692 w697]
                          tunnel: w684 -> [_ w696]
                          tunnel: [w689 w695] -> w683
                          tunnel: w681 -> [w690 w694]
                          tunnel: [w688 w694] -> w680
                          tunnel: w679 -> [w691 _]
                          tunnel: w678 -> [w687 _]
                          frame "Array" {
                            n135 = call "JSON text to Variant.vi"("LVClass Serializer"=w687, "error in (no error)"=w690, "Data Type"=w691, "Offset"=w692, "JSON"=w693) -> ("error out"=w688:errorcluster, "Variant out"=w689:variant)  [unwired: 5 in]
                          }
                          frame "String", Default {
                            n136 = call "String Subset.vi"("Offset past End"=w696, "Start offset"=w697, "JSON"=w698) -> ("substring"=w695:string)  [unwired: 2 in]
                          }
                        }
                      }
                    }
                  }
                }
              }
            }
            frame Error {
              # "Issue 40"
            }
          }
          n137 = call "Array of Variants to Cluster.vi"("Array of Variants"=w618) -> ("Cluster of Variants"=w608:variant)  [unwired: 10 in]
          n138 = Merge Errors(w604, w607) -> (w617:errorcluster)
        }
        frame "JSON Array" {
          n139 = Variant To Data(error in=w722, type=variant[] [], Variant=w724) -> (data=w719:variant[], error out=w720:errorcluster)
          n140 = call "Possible Ragged Array.vi"("Array"=w719) -> ("Ragged Array posible"=w716:bool)  [unwired: 10 in]
          n141 = case shown="False" w716 {
            tunnel: [w738 w778] -> w721
            tunnel: w717 -> [w726 w781]
            tunnel: w720 -> [w737 w779]
            tunnel: w719 -> [w730 w784]
            tunnel: w718 -> [w729 w782]
            tunnel: [w727 w776] -> w715
            tunnel: w714 -> [w736 _]
            tunnel: w713 -> [w725 w775]
            frame False {
              # "First Cluster Element Unnamed"
              n142 = Index Array(array=w730) -> (element=w735:variant)  [unwired: 1 in]
              n143 = call <vilib>:"Get Type Information.vi"("variant"=w735) -> ("name"=w732:string, "type"=w733:T1)  [unwired: 6 in, 3 out]
              n144 = case shown="\"String\", \"Array\"" w733 {
                tunnel: w732 -> [w739 w741]
                tunnel: [w739 w740] -> w734
                frame Default {
                }
                frame "String", "Array" {
                  n145 = call "Remove JSON Tag.vi"("Name"=w741) -> ("Name (tag stripped)"=w740:string)  [unwired: 9 in, 1 out]
                }
              }
              n146 = Empty String/Path?(string/path=w734) -> (empty?=w731:bool)
              n147 = case shown="True" w731 {
                tunnel: [w745 w756] -> w738
                tunnel: w737 -> [w744 w751]
                tunnel: w736 -> [w743 _]
                tunnel: [w742 w753] -> w728
                tunnel: w730 -> [w742 w755]
                tunnel: w729 -> [_ w754]
                tunnel: w726 -> [_ w752]
                tunnel: w725 -> [_ w749]
                frame False {
                  n148 = Format Into String(w743) -> (resulting string=w746:string)  [unwired: 3 in, 1 out]
                  n149 = call "Format Error.vi"("error code (402842)"=402844, "error in (no error)"=w744, "message part 2"=w746, "error message"="Cannot Get Array as a Cluster: " ("format string")) -> ("error out"=w745:errorcluster)  [unwired: 7 in]
                }
                frame True {
                  # "Unnamed cluster elements\n--> JSON Array"
                  n150 = call "Get Array Elements.vi"("error in (no error)"=w751, "Offset"=w752, "JSON"=w754) -> ("error out"=w750:errorcluster, "<JSON>"=w757:string[])  [unwired: 6 in, 1 out]
                  n151 = for {
                    tunnel: w755 -> [w766] mode=indexing
                    tunnel: w750 -> [w764]
                    tunnel: [w763] -> w758 mode=indexing
                    tunnel: [w765] -> w753 mode=indexing
                    tunnel: w757 -> [w762]
                    tunnel: w749 -> [w759]
                    i -> [w760]
                    n152 = Index Array(array=w762, index=w760) -> (element=w761:string)
                    n153 = case shown="Default" w761 {
                      selector: w761 -> [_ w770]
                      tunnel: w766 -> [w768 w774]
                      tunnel: [w768 w773] -> w765
                      tunnel: w764 -> [w767 w772]
                      tunnel: [w767 w771] -> w763
                      tunnel: w759 -> [_ w769]
                      frame "" {
                      }
                      frame Default {
                        n154 = call "JSON text to Variant.vi"("LVClass Serializer"=w769, "error in (no error)"=w772, "Data Type"=w774, "JSON"=w770) -> ("error out"=w771:errorcluster, "Variant out"=w773:variant)  [unwired: 6 in]
                      }
                    }
                  }
                  n155 = Merge Errors(w758) -> (w756:errorcluster)
                }
              }
              n156 = call "Array of Variants to Cluster.vi"("Array of Variants"=w728) -> ("Cluster of Variants"=w727:variant)  [unwired: 10 in]
            }
            frame True {
              # "Let a JSON Array be valid for an Array as sole element in a Cluster, as this is a way of doing \"Ragged\" arrays in LabVIEW."
              n157 = Index Array(array=w784) -> (element=w783:variant)  [unwired: 1 in]
              n158 = call "JSON text to Variant.vi"("LVClass Serializer"=w775, "error in (no error)"=w779, "Data Type"=w783, "Offset"=w781, "JSON"=w782) -> ("error out"=w778:errorcluster, "Variant out"=w780:variant)  [unwired: 5 in]
              n159 = Build Array(w780) -> (w777:variant[])
              n160 = call "Array of Variants to Cluster.vi"("Array of Variants"=w777) -> ("Cluster of Variants"=w776:variant)  [unwired: 10 in]
            }
          }
        }
      }
    }
    frame "Variant", "LV Variant" {
      # "Unwrap and rewrap"
      n161 = Variant To Data(error in=w794, type=variant, Variant=w795) -> (data=w786:variant, error out=w791:errorcluster)
      n162 = call "JSON text to Variant.vi"("LVClass Serializer"=w785, "error in (no error)"=w791, "Data Type"=w786, "Offset"=w789, "JSON"=w790) -> ("error out"=w787:errorcluster, "Variant out"=w788:variant)  [unwired: 5 in]
      n163 = To Variant(anything=w788) -> (Variant=w792:variant)
    }
    frame "LabVIEW Class Instance" {
      n164 = Variant To Data(error in=w804, type=refnum<class> refnum ("LabVIEW Object"), Variant=w806) -> (data=w802:refnum<class>, error out=w805:errorcluster)
      n165 = Not Equal?(x=w798, y=refnum<class "JSONtext LVClass Serializer.lvclass"> refnum) -> (x != y?=w796:bool)
      n166 = case shown="False" w796 {
        tunnel: w798 -> [_ w820]
        tunnel: w807 -> [w813 w819]
        tunnel: w805 -> [w809 w818]
        tunnel: w802 -> [w808 w817]
        tunnel: [w811 w816] -> w801
        tunnel: [w810 w815] -> w800
        tunnel: w799 -> [w812 w814]
        frame False {
          n167 = call "JSON to LVObject.vi"("error in (no error)"=w809, "JSON"=w813, "Offset of first non-whitespace"=w812, "LabVIEW Object in"=w808) -> ("error out"=w810:errorcluster, "LabVIEW Object out"=w811:refnum<class>)  [unwired: 6 in]
        }
        frame True {
          # "Issue #56 Way of providing alternate format\nof LVObjects"
          n168 = call-dynamic "JSON to LVObject.vi"("JSONtext LVClass Serializer in"=w820, "error in (no error)"=w818, "Object Type"=w817, "Offset"=w814, "JSON"=w819) -> ("error out"=w815:errorcluster, "Object"=w816:refnum<class>)  [unwired: 5 in]
        }
      }
    }
  }
  "Variant out" <- w7
  "error out" <- w9
